vi "Train.vi"(6 "Parallel Instances (8)":i32=8, 7 "Queue in":refnum<queue>, 8 "error in (no error)":errorcluster, 9 "Progress ref in":refnum<vi>, 10 "File Data Array":T1[](array[typedef]), 11 "AbstractModel in":refnum<class "AbstractModel.lvclass">) -> (0 "error out":errorcluster, 3 "AbstractModel out":refnum<class "AbstractModel.lvclass">)   [LabVIEW 2024, in "AbstractModel.lvclass"]
uses:
  AbstractModel.lvclass
  AbstractModel.lvclass/AbstractModel.ctl
  File Metadata.ctl
  Node.ctl
  Source to Sink Array.ctl
  File Data.ctl
  Indexer Action.ctl
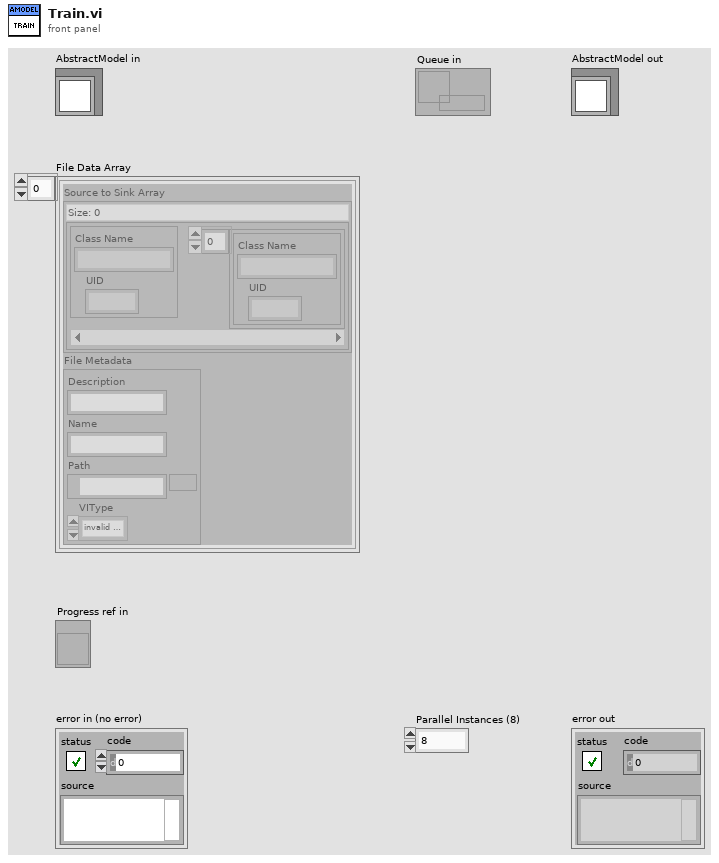
[diagram p1: front panel]
types:
  T1 = typedef "File Data.ctl" = cluster{"Source to Sink Array":T2, "File Metadata":T4}
  T2 = typedef "Source to Sink Array.ctl" = map{T3, T3[]}
  T3 = typedef "Node.ctl" = cluster{"Class Name":string, "UID":i32}
  T4 = typedef "File Metadata.ctl" = cluster{"Description":string, "Name":string, "Path":path, "VIType":enum32{"invalid VI type", "Standard VI", "Control VI", "Global VI", "Polymorphic VI", "Configuration VI", "SubSystem", "Facade VI", "Method VI", "Statechart Diagram VI"}}
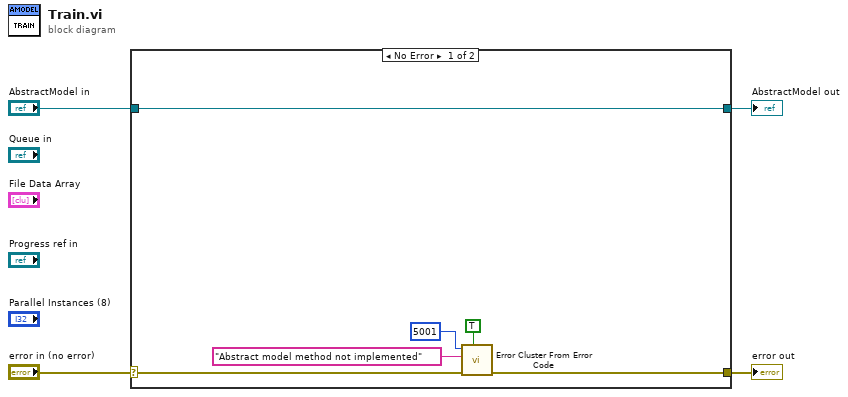
[diagram p0: block diagram]
diagram:
  n1 = case shown="No Error" "error in (no error)" {
    selector: "error in (no error)" -> [w9 w12]
    tunnel: [w8 w12] -> w3
    tunnel: [w10 w11] -> w1
    tunnel: "AbstractModel in" -> [w10 w11]
    frame No Error {
      n2 = call <vilib>:"Error Cluster From Error Code.vi"("show call chain? (False)"=TRUE, "error in (no error)"=w9, "error message (\"\")"="Abstract model method not implemented" ("error message (\"\")"), "error code (0)"=5001) -> ("error out"=w8:errorcluster)  [unwired: 5 in]
    }
    frame Error {
    }
  }
  "error out" <- w3
  "AbstractModel out" <- w1
